vi "Get_MAC_Address.vi"(5 "error in (no error)":errorcluster) -> (0 "error out":errorcluster, 2 "MAC Address Hex":i32, 3 "MAC Address":string)   [LabVIEW 2013]
uses:
  <vilib>/Utility/error.llb/whitespace.ctl
panel:
  out "result string":string
  out "standard output":string
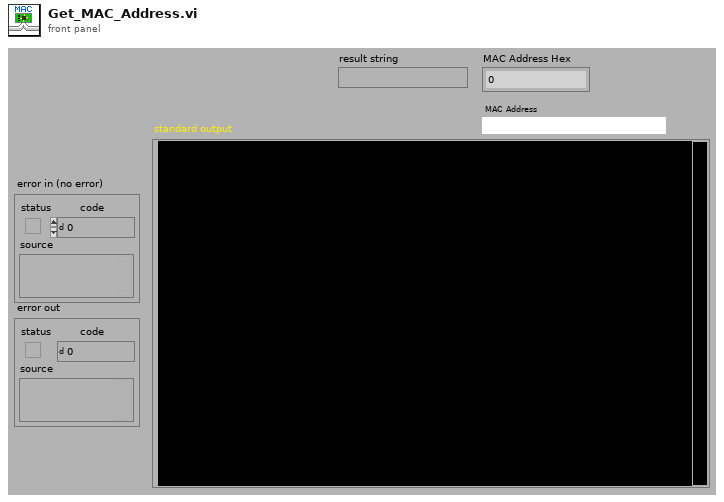
[diagram p1: front panel]
types:
  T1 = typedef "whitespace.ctl" = u16
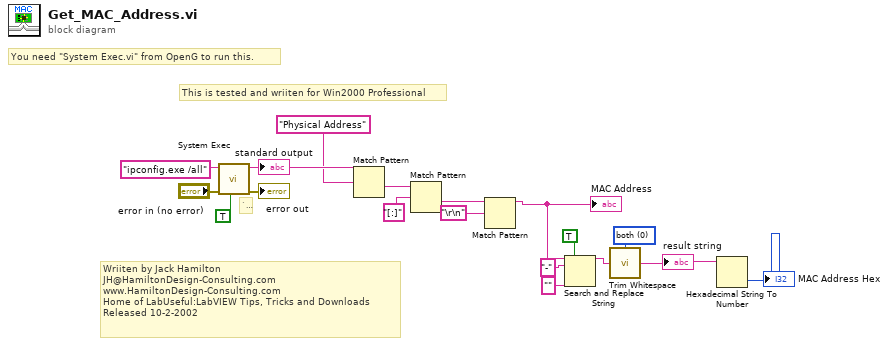
[diagram p0: block diagram]
diagram:
  w3 = T1 0 items=["both", "start of string", "end of string"] ("location (both)")
  # "```"
  # "You need \"System Exec.vi\" from OpenG to run this."
  # "Wriiten by Jack Hamilton\nJH@HamiltonDesign-Consulting.com\nwww.HamiltonDesign-Consulting.com\nHome of LabUseful:LabVIEW Tips, Tricks and Downloads\nReleased 10-2-2002"
  # "This is tested and wriiten for Win2000 Professional"
  n1 = call <vilib>:"System Exec.vi"("run minimized? (F)"=TRUE, "error in (no error)"="error in (no error)", "command line"="ipconfig.exe /all") -> ("error out"=→"error out":errorcluster, "standard output"=w17:string)  [unwired: 3 in, 4 out]
  "standard output" <- w17
  n2 = Match Pattern(string=w17, regular expression="Physical Address") -> (after substring=w13:string)  [unwired: 4 out]
  n3 = Match Pattern(string=w13, regular expression="[:]") -> (after substring=w11:string)  [unwired: 4 out]
  n4 = Match Pattern(string=w11, regular expression="\r\n") -> (before substring=w8:string)  [unwired: 4 out]
  "MAC Address" <- w8
  n5 = Search and Replace String(replace all?=TRUE ("replace all? (F)"), input string=w8, search string="-", replace string="" ("replace string (\"\")")) -> (result string=w4:string)  [unwired: 1 in, 6 out]
  n6 = call <vilib>:"Trim Whitespace.vi"("string"=w4, "location (both)"=w3) -> ("trimmed string"=w2:string)
  "result string" <- w2
  n7 = Hexadecimal String To Number(string=w2) -> (number=→"MAC Address Hex":u32)  [unwired: 3 out]
